vi "PWM Init.vi"(10 "pConfig":T1, 11 "DevHandle":i32) -> (2 "pConfig out":T1, 3 "function return":i32)   [LabVIEW 2010, in "usb2pwm.lvlib"]
doc: "int WINAPI PWM_Init(int DevHandle, PPWM_CONFIG pConfig);"
uses:
  usb2pwm.lvlib
  USB2XXX/trunk/USB2XXX/USB2XXX/vs2019/Release/USB2XXX.dll
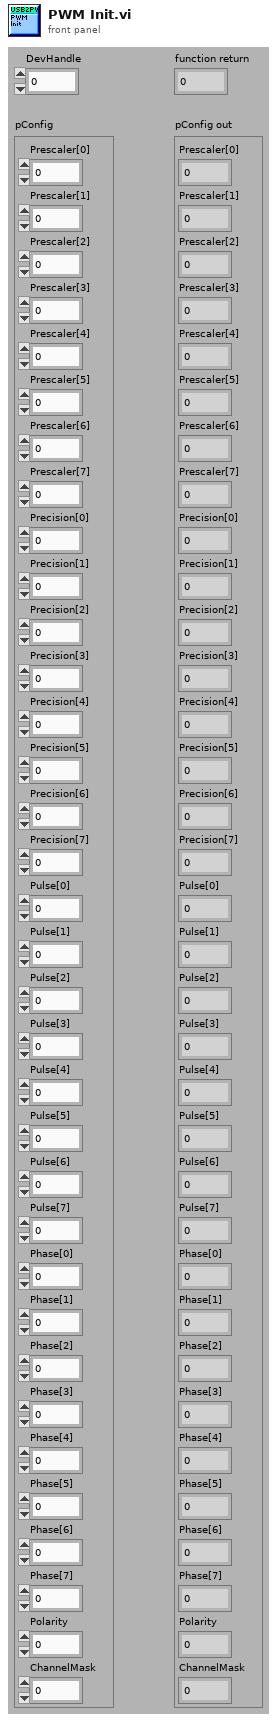
[diagram p1: front panel]
types:
  T1 = cluster{"Prescaler[0]":u16, "Prescaler[1]":u16, "Prescaler[2]":u16, "Prescaler[3]":u16, "Prescaler[4]":u16, "Prescaler[5]":u16, "Prescaler[6]":u16, "Prescaler[7]":u16, "Precision[0]":u16, "Precision[1]":u16, "Precision[2]":u16, "Precision[3]":u16, "Precision[4]":u16, "Precision[5]":u16, "Precision[6]":u16, "Precision[7]":u16, "Pulse[0]":u16, "Pulse[1]":u16, "Pulse[2]":u16, "Pulse[3]":u16, "Pulse[4]":u16, "Pulse[5]":u16, "Pulse[6]":u16, "Pulse[7]":u16, "Phase[0]":u16, "Phase[1]":u16, "Phase[2]":u16, "Phase[3]":u16, "Phase[4]":u16, "Phase[5]":u16, "Phase[6]":u16, "Phase[7]":u16, "Polarity":u8, "ChannelMask":u8}
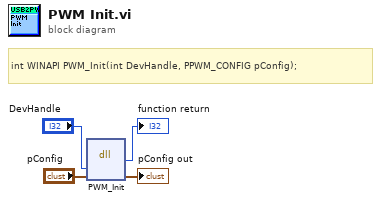
[diagram p0: block diagram]
diagram:
  # "int WINAPI PWM_Init(int DevHandle, PPWM_CONFIG pConfig);"
  n1 = dll-call lib="E:/Projects/USB2XXX/trunk/USB2XXX/USB2XXX/vs2019/Release/USB2XXX.*" fn="PWM_Init"("DevHandle"="DevHandle", "pConfig"="pConfig") -> (→"function return":i32, "pConfig"=→"pConfig out":T1)  [unwired: 4 in, 2 out]
